vi "error module.vi"(8 "error in (no error)":errorcluster, 10 "cluster 2":T1, 11 "Enum":T2=enum."Report Errors") -> (0 "error out":errorcluster)   [LabVIEW 2019]
uses:
  error module commands.ctl
  Main VI references.ctl
  main queue data type.ctl
  top level commands.ctl
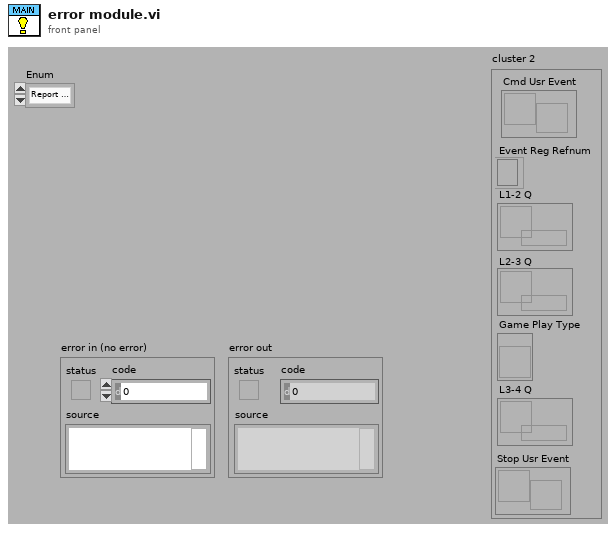
[diagram p1: front panel]
types:
  T1 = typedef "Main VI references.ctl" = cluster{"Cmd Usr Event":refnum<user-event>, "Event Reg Refnum":refnum<event-registration>, "L1-2 Q":refnum<queue>, "L2-3 Q":refnum<queue>, "Game Play Type":refnum<vi>, "L3-4 Q":refnum<queue>, "Stop Usr Event":refnum<user-event>}
  T2 = typedef "error module commands.ctl" = enum16{"Cleanup References", "Set References", "Report Errors", "Process Errors"}
  T3 = typedef "main queue data type.ctl" = cluster{"Command":T4, "Data":variant}
  T4 = typedef "top level commands.ctl" = enum16{"Idle", "Set Cube Orientation", "Get Cube Orientation", "Go to Face", "Solve", "Test", "Randomize", "Game Play Type", "Stop", "rotate Cube"}
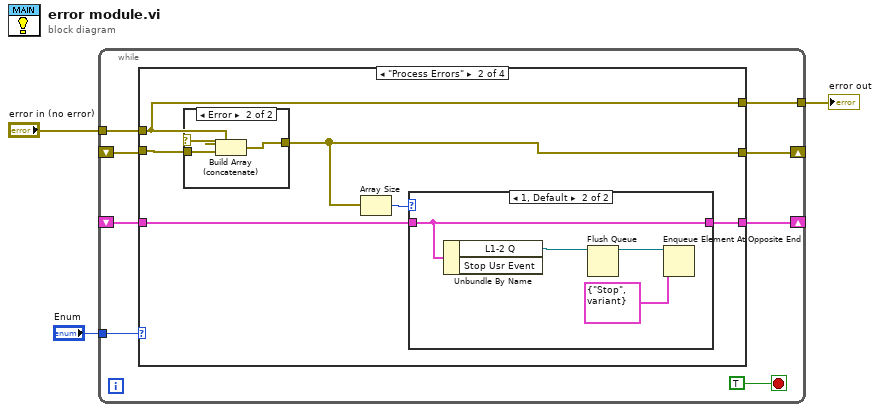
[diagram p0: block diagram]
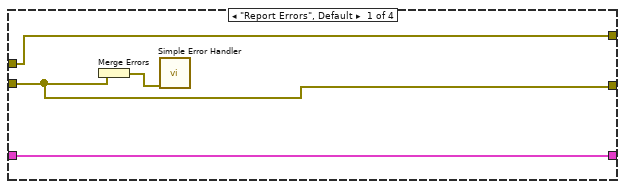
[diagram p2: hidden frame]
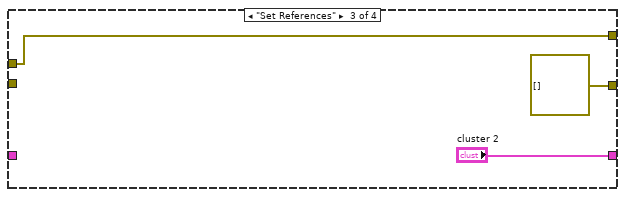
[diagram p5: hidden frame]
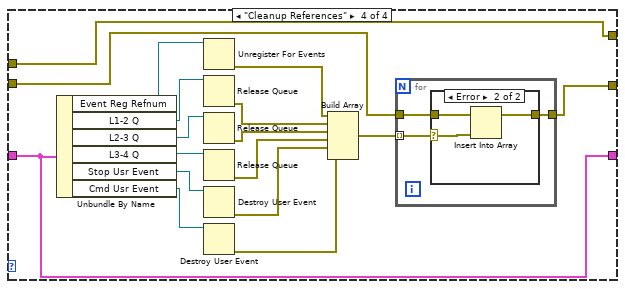
[diagram p6: hidden frame]
diagram:
  n1 = while {
    tunnel: "Enum" -> [w10]
    shift-right: [w9] -> _
    shift-left: _ -> [w8]
    shift-right: [w7] -> _
    shift-left: _ -> [w6]
    tunnel: "error in (no error)" -> [w5]
    tunnel: [w4] -> w1
    stop <- TRUE stop-if-true
    n2 = case shown="\"Process Errors\"" w10 {
      tunnel: [w14 w19 "cluster 2" w44] -> w9
      tunnel: w8 -> [w14 w18 _ w44]
      tunnel: w6 -> [w13 w21 _ w35]
      tunnel: [w13 w16 errorcluster[] [] w34] -> w7
      tunnel: w5 -> [w12 w17 w32 w36]
      tunnel: [w12 w17 w32 w36] -> w4
      frame "Report Errors", Default {
        n3 = Merge Errors(w13) -> (w15:errorcluster)
        n4 = call <vilib>:"Simple Error Handler.vi"("error in (no error)"=w15) -> ()  [unwired: 4 in, 5 out]
      }
      frame "Process Errors" {
        n5 = case shown="Error" w17 {
          selector: w17 -> [_ w30]
          tunnel: [w27 w29] -> w16
          tunnel: w21 -> [w27 w28]
          frame No Error {
          }
          frame Error {
            n6 = Build Array (concatenate)(w30, w28) -> (w29:errorcluster[])
          }
        }
        n7 = Array Size(array=w16) -> (size(s)=w20:i32)
        n8 = case shown="1, Default" w20 {
          tunnel: [w22 w23] -> w19
          tunnel: w18 -> [w22 w23]
          frame 0 {
          }
          frame 1, Default {
            n9 = Unbundle By Name(w23) -> ("L1-2 Q"=w26:refnum<queue>)  [unwired: 1 out]
            n10 = Flush Queue(queue=w26) -> (queue out=w25:refnum<queue>)  [unwired: 1 in, 2 out]
            n11 = Enqueue Element At Opposite End(queue=w25, element=T3 {"Command"=enum."Stop", "Data"=variant}) -> ()  [unwired: 2 in, 3 out]
          }
        }
      }
      frame "Set References" {
      }
      frame "Cleanup References" {
        n12 = Unbundle By Name(w44) -> ("Event Reg Refnum"=w50:refnum<event-registration>, "L1-2 Q"=w49:refnum<queue>, "L2-3 Q"=w48:refnum<queue>, "L3-4 Q"=w47:refnum<queue>, "Stop Usr Event"=w46:refnum<user-event>, "Cmd Usr Event"=w45:refnum<user-event>)
        n13 = Unregister For Events(event registration refnum=w50) -> (error out=w43:errorcluster)  [unwired: 1 in]
        n14 = Release Queue(queue=w49) -> (error out=w42:errorcluster)  [unwired: 2 in, 2 out]
        n15 = Release Queue(queue=w48) -> (error out=w41:errorcluster)  [unwired: 2 in, 2 out]
        n16 = Release Queue(queue=w47) -> (error out=w40:errorcluster)  [unwired: 2 in, 2 out]
        n17 = Destroy User Event(user event=w46) -> (error out=w39:errorcluster)  [unwired: 1 in]
        n18 = Destroy User Event(user event=w45) -> (error out=w38:errorcluster)  [unwired: 1 in]
        n19 = Build Array(w43, w42, w41, w40, w39, w38) -> (w37:errorcluster[])
        n20 = for {
          tunnel: w37 -> [w53] mode=indexing
          tunnel: w35 -> [w52]
          tunnel: [w51] -> w34
          n21 = case shown="Error" w53 {
            selector: w53 -> [_ w57]
            tunnel: w52 -> [w54 w56]
            tunnel: [w54 w55] -> w51
            frame No Error {
            }
            frame Error {
              n22 = Insert Into Array(array=w56, new element=w57) -> (w55:errorcluster[])  [unwired: 1 in]
            }
          }
        }
      }
    }
  }
  "error out" <- w1
